vi "Append Image HF.vi"(0 "PDF Report IN":T24(xcontrol), 2 "Header or footer":T1={"Start at page"=1, "H/F Alignment"=enum."CENTER - middle", "Path"=path "", "Image (%)"=100.0, "Link"=""}, 11 "error in (no error)":errorcluster, 13 "Position":T3) -> (4 "PDF Report OUT":T24(xcontrol), 15 "error out":errorcluster)   [LabVIEW 2013]
doc: "Appends an <B>image</B> in a column header (or footer). You can use this polymorphic VI to append a colomn to a header (or footer). The data type you wire to the <B>Header or footer</B> input determines the polymorphic instance to use.\n\nThe header (or footer) can be divided up into three columns. Each column has the same width. The number of header (or footer) that you add determines the number of columns.\n\n<B>FRANÇAIS</B>\nAjoute une <B>image</B> dans une colonne d'un en-tête (ou d'un pied de page). Vous pouvez utiliser ce VI polymorphique pour ajouter une colonne à un en-tête (ou un pied de page). Le type de variable que vous reliez au terminal <B>Header or footer</B> détermine l'instance polymorphique à utiliser.\n\nL'en-tête (ou le pied de page) peut être divisé en un maximum de trois colonnes. Chaque colonne a la même largeur. Le nombre d'en-têtes (ou de pieds de page) que vous ajoutez détermine le nombre de colonnes.\n\n\n\nVersion 1.0\nDeveloped by Jean-Marc Simard\nCopyright © 2010, Exaprom Inc.\nAll rights reserved.\nLicense: BSD\n\nWith iTextSharp 4.1.6 (http://itextsharp.sourceforge.net)\nunder Mozilla Public License Version 1.1\n(http://www.mozilla.org/MPL/MPL-1.1.html)"
uses:
  Controls/PDF Report Xcontrol/PDF Report.xctl
  Controls/Header or Footer.ctl
  Controls/Header or Footer  Image cluster.ctl
  Controls/H F Alignment.ctl
  Controls/Header Footer cluster.ctl
  Controls/Header Footer Type.ctl
  Controls/Header footer horiz alignment.ctl
  Controls/Cell Vertical alignment.ctl
  Controls/Page number.ctl
  Controls/Font cluster.ctl
  Controls/Font size.ctl
  Controls/Font color.ctl
  Controls/Header Footer Line.ctl
  C:/Users/MaxCorp/Documents/GitHub/TopView/DLL/itextsharp.dll
  DLL/itextsharp.dll
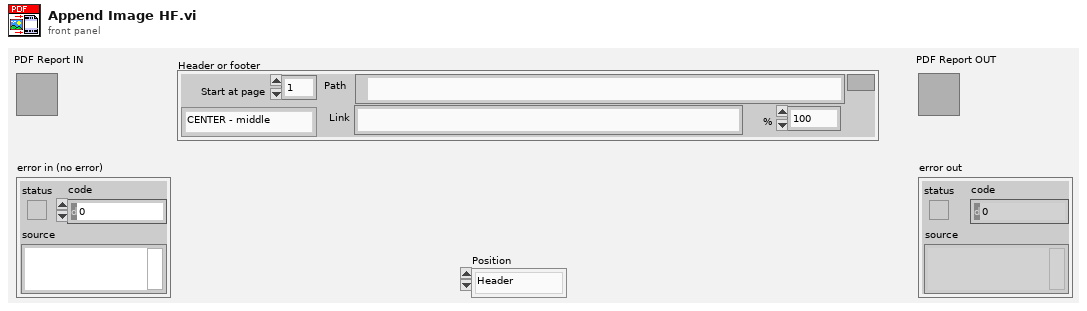
[diagram p1: front panel]
types:
  T1 = typedef "Header or Footer  Image cluster.ctl" = cluster{"Start at page":i32, "H/F Alignment":T2, "Path":path, "Image (%)":sgl, "Link":string}
  T2 = typedef "H F Alignment.ctl" = enum16{"LEFT - top", "LEFT - middle", "LEFT - bottom", "CENTER - top", "CENTER - middle", "CENTER - bottom", "RIGHT - top", "RIGHT - middle", "RIGHT - bottom", ""}
  T3 = typedef "Header or Footer.ctl" = enum16{"Header", "Footer"}
  T4 = typedef "Font cluster.ctl" = cluster{"Name":string, "Size":T5, "Color":T6, "Style":cluster{"Bold":bool, "Italic":bool, "Underline":bool, "Strikeout":bool}}
  T5 = typedef "Font size.ctl" = sgl
  T6 = typedef "Font color.ctl" = u32
  T7 = typedef "Unit.ctl" = enum16{"inch", "mm"}
  T8 = typedef "Paragraphe cluster.ctl" = cluster{" Aligment":T9, "Line spacing":T10}
  T9 = typedef "Texte alignement.ctl" = enum16{"Select", "CENTER", "JUSTIFY", "LEFT", "RIGHT"}
  T10 = typedef "Line spacing.ctl" = enum16{"Select", "1.0", "1.5", "2.0"}
  T11 = typedef "Page dimensions.ctl" = cluster{"Start at page":i32, "Orientation":T12, "widht":sgl, "height":sgl, "Margin left":sgl, "Margin right":sgl, "Margin top":sgl, "Margin bottom":sgl}
  T12 = typedef "Page Orientation.ctl" = enum16{"Portrait", "Landscape"}
  T13 = typedef "Image or Table Caption.ctl" = cluster{"Caption":string, "Separator":string, "Position":enum16{"Above", "Below"}}
  T14 = typedef "Header Footer [ ].ctl" = T15[]
  T15 = typedef "Header Footer cluster.ctl" = cluster{"Start page":i32, "Type":T16, "Alignment":T17, "Vertical Alignement":T18, "Image (%)":sgl, "Page #":T19, "Text":string, "Path":string, "Font":T4, "Font refnum":refnum<k24>, "Line":cluster{"Line":T20, "Thickness (points)":sgl, "Colour":T6}}
  T16 = typedef "Header Footer Type.ctl" = enum16{"Select", "Text", "Text + hyperlink", "Page number", "Image", "Image + hyperlink"}
  T17 = typedef "Header footer horiz alignment.ctl" = enum16{"Left", "Center", "Right"}
  T18 = typedef "Cell Vertical alignment.ctl" = enum16{"TOP", "MIDDLE", "BOTTOM"}
  T19 = typedef "Page number.ctl" = cluster{"Text 1":string, "Text 2":string, "Text 3":string}
  T20 = typedef "Header Footer Line.ctl" = enum16{"No line", "Horizontal line"}
  T21 = typedef "Watermark cluster2.ctl" = cluster{"Show? (F)":bool, "Type":enum16{"Image", "Text"}, "Opacity (%)":sgl, "Rotate(°)":sgl, "Position":cluster{"Position":T22, "X":sgl, "Y":sgl}, "Image path":path, "Scaled(%)":sgl, "Image refnum":refnum<k24>, "Text":string, "Font":cluster{"Name":string, "Size":T5, "Color":T6}, "Font refnum":refnum<k24>, "Alignment":T17, "Automatic":bool}
  T22 = typedef "Watermark Position.ctl" = enum16{"Absolute", "Center (page)", "Center (text section)"}
  T23 = typedef "System Fonts.ctl" = cluster{"Font name [ ]":string[], "Font and file names [ ]":cluster{"Font name":string, "File name":string}[]}
  T24 = cluster{"Document":refnum<k24>, "Writer":refnum<k24>, "Default Font":refnum<k24>, "Default Font cluster":T4, "Path":path, "Unit (default = mm)":T7, "Paragraphe cluster":T8, "Pages dimensions [ ]":T11[], "Captions":cluster{"Image":T13, "Image counter":u16, "Table":T13, "Table counter":u16, "Font":T4}, "Header":T14, "Footer":T14, "Watermark ":T21, "Actual VI name":string, "System Fonts":T23}
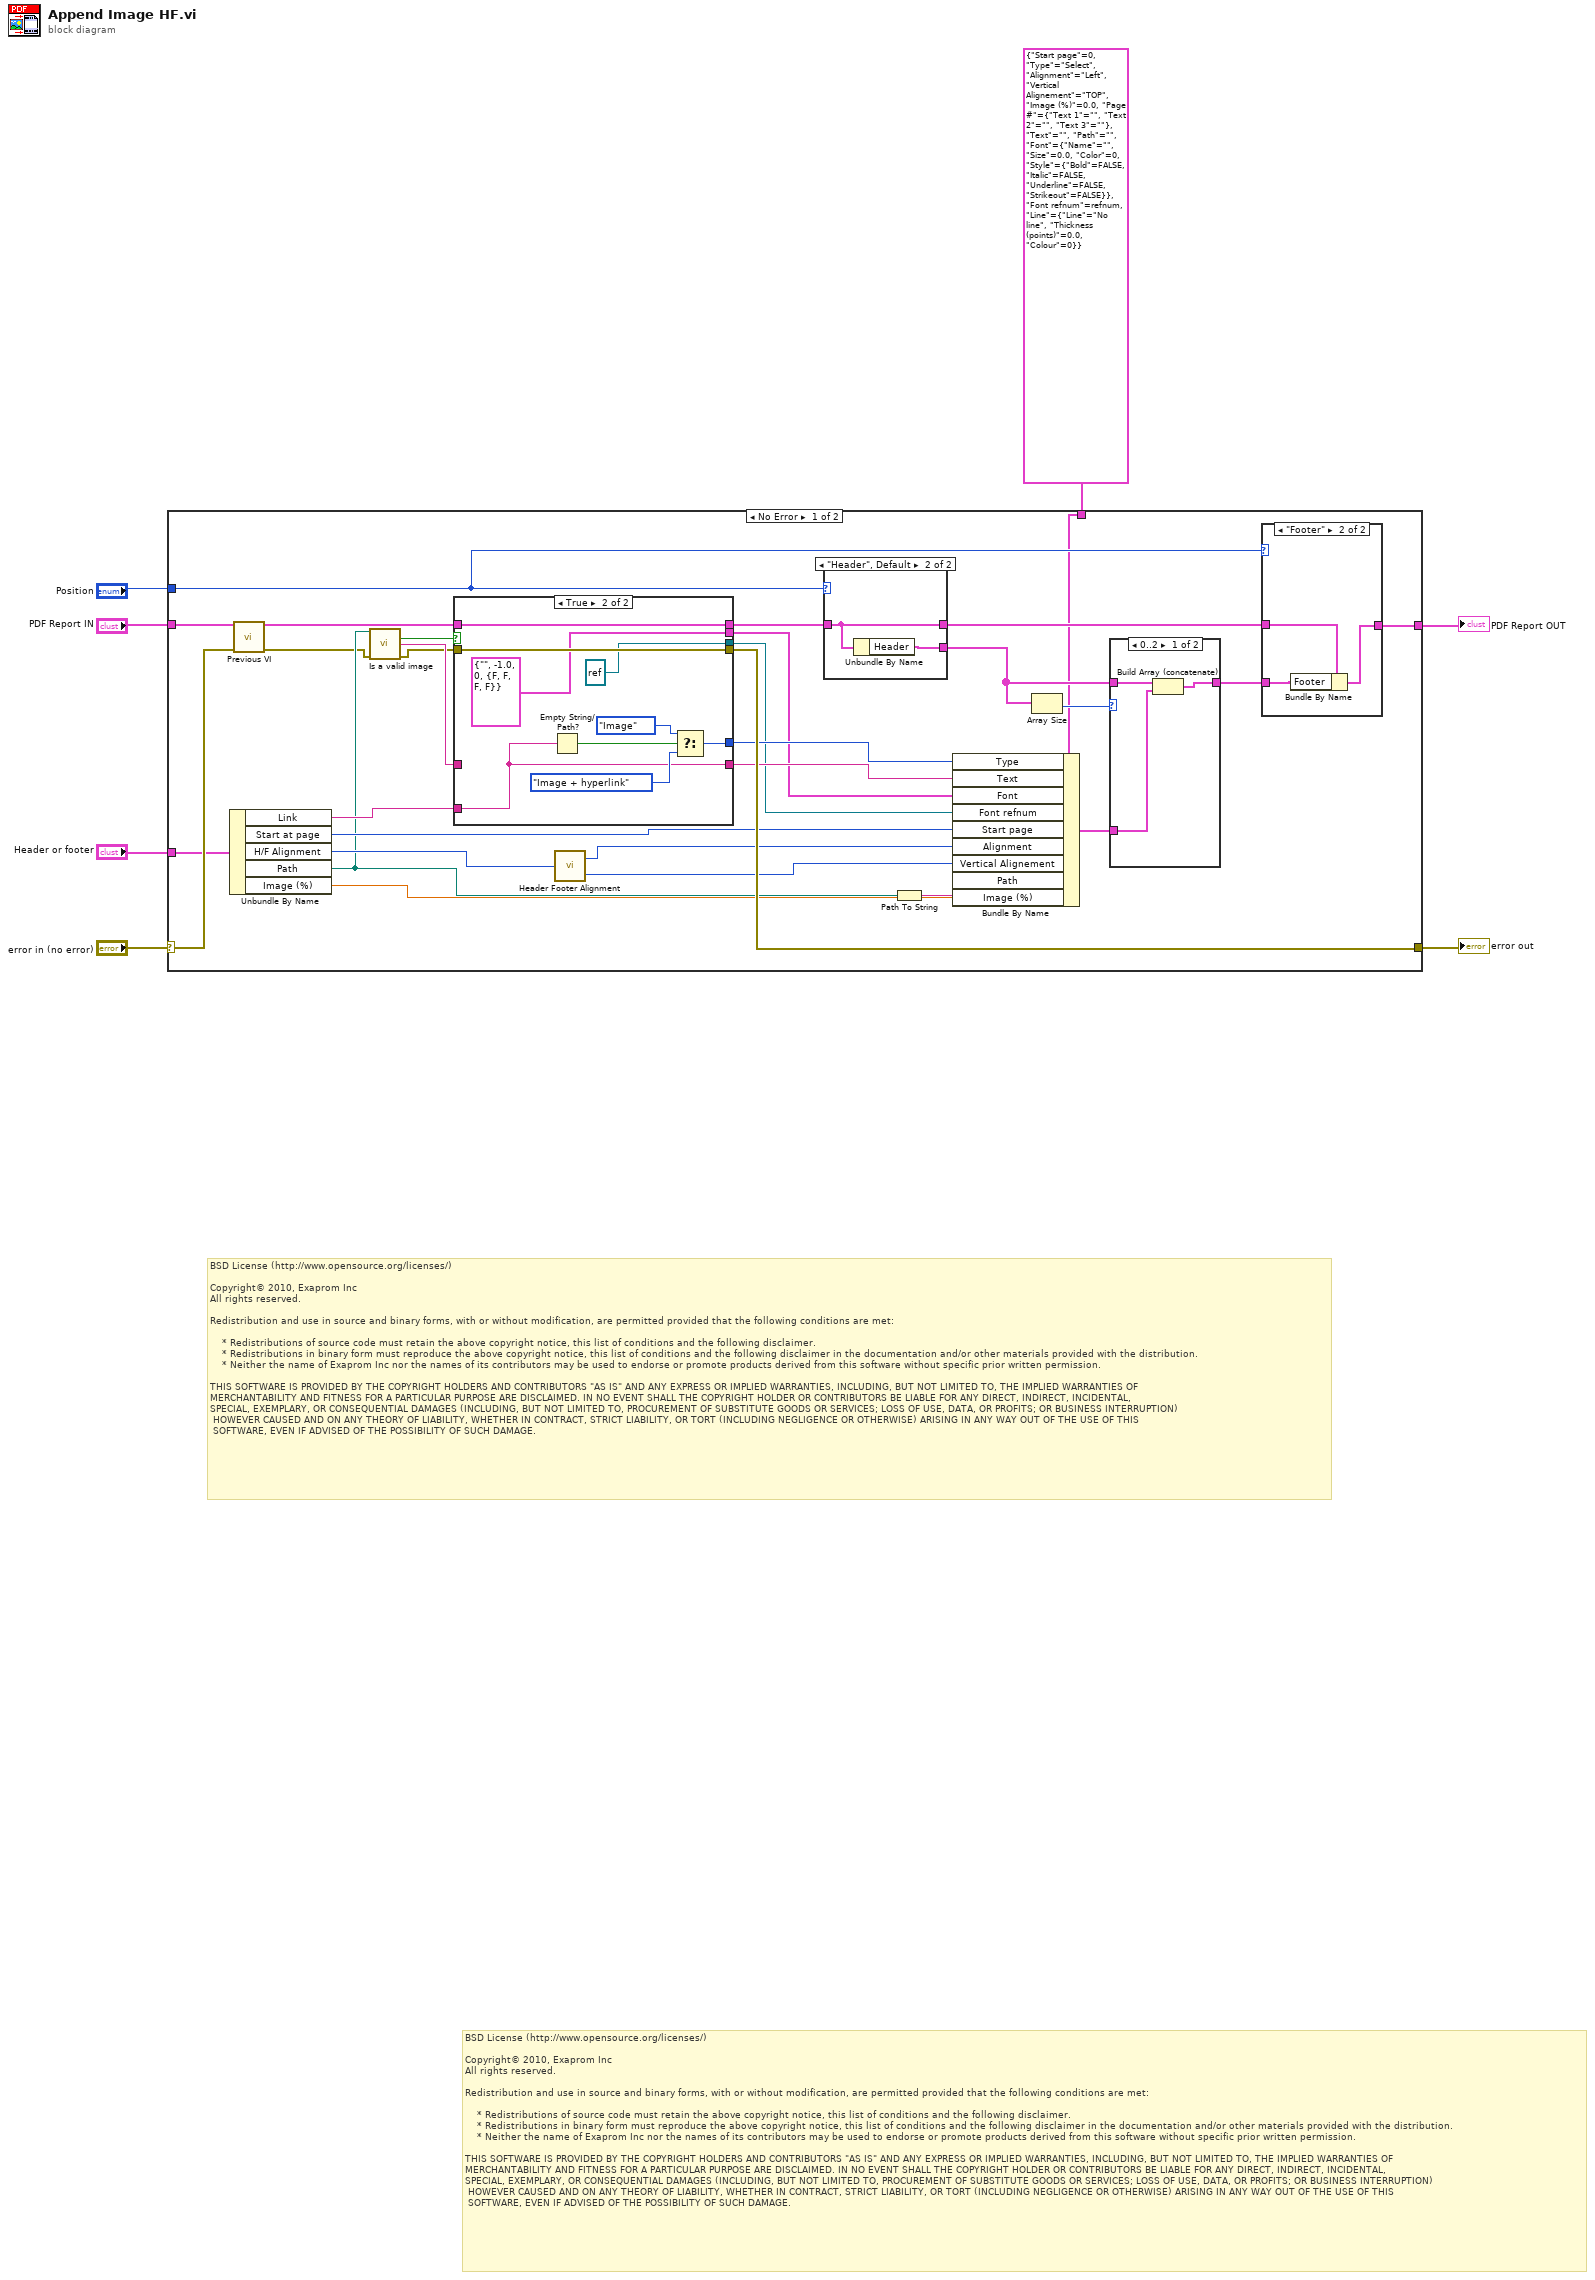
[diagram p0: block diagram]
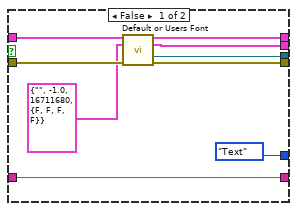
[diagram p2: hidden frame]
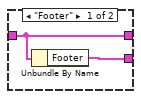
[diagram p4: hidden frame]
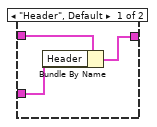
[diagram p5: hidden frame]
diagram:
  # "BSD License (http://www.opensource.org/licenses/)\n\nCopyright© 2010, Exaprom Inc\nAll rights reserved.\n\nRedistribution and use in source and binary forms, with or without modification, are permitted provided that the following conditions are met:\n\n    * Redistributions of source code must retain the above copyright notice, this list of conditions and the following disclaimer.\n    * Redistributions in binary form must reproduce the above copyright notice, this list of conditions and the following disclaimer in the documentation and/or other materials provided with the distribution.\n    * Neither the name of Exaprom Inc nor the names of its contributors may be used to endorse or promote products derived from this software without specific prior written permission.\n\nTHIS SOFTWARE IS PROVIDED BY THE COPYRIGHT HOLDERS AND CONTRIBUTORS \"AS IS\" AND ANY EXPRESS OR IMPLIED WARRANTIES, INCLUDING, BUT NOT LIMITED TO, THE IMPLIED WARRANTIES OF \nMERCHANTABILITY AND FITNESS FOR A PARTICULAR PURPOSE ARE DISCLAIMED. IN NO EVENT SHALL THE COPYRIGHT HOLDER OR CONTRIBUTORS BE LIABLE FOR ANY DIRECT, INDIRECT, INCIDENTAL,\nSPECIAL, EXEMPLARY, OR CONSEQUENTIAL DAMAGES (INCLUDING, BUT NOT LIMITED TO, PROCUREMENT OF SUBSTITUTE GOODS OR SERVICES; LOSS OF USE, DATA, OR PROFITS; OR BUSINESS INTERRUPTION)\n HOWEVER CAUSED AND ON ANY THEORY OF LIABILITY, WHETHER IN CONTRACT, STRICT LIABILITY, OR TORT (INCLUDING NEGLIGENCE OR OTHERWISE) ARISING IN ANY WAY OUT OF THE USE OF THIS\n SOFTWARE, EVEN IF ADVISED OF THE POSSIBILITY OF SUCH DAMAGE."
  # "BSD License (http://www.opensource.org/licenses/)\n\nCopyright© 2010, Exaprom Inc\nAll rights reserved.\n\nRedistribution and use in source and binary forms, with or without modification, are permitted provided that the following conditions are met:\n\n    * Redistributions of source code must retain the above copyright notice, this list of conditions and the following disclaimer.\n    * Redistributions in binary form must reproduce the above copyright notice, this list of conditions and the following disclaimer in the documentation and/or other materials provided with the distribution.\n    * Neither the name of Exaprom Inc nor the names of its contributors may be used to endorse or promote products derived from this software without specific prior written permission.\n\nTHIS SOFTWARE IS PROVIDED BY THE COPYRIGHT HOLDERS AND CONTRIBUTORS \"AS IS\" AND ANY EXPRESS OR IMPLIED WARRANTIES, INCLUDING, BUT NOT LIMITED TO, THE IMPLIED WARRANTIES OF \nMERCHANTABILITY AND FITNESS FOR A PARTICULAR PURPOSE ARE DISCLAIMED. IN NO EVENT SHALL THE COPYRIGHT HOLDER OR CONTRIBUTORS BE LIABLE FOR ANY DIRECT, INDIRECT, INCIDENTAL,\nSPECIAL, EXEMPLARY, OR CONSEQUENTIAL DAMAGES (INCLUDING, BUT NOT LIMITED TO, PROCUREMENT OF SUBSTITUTE GOODS OR SERVICES; LOSS OF USE, DATA, OR PROFITS; OR BUSINESS INTERRUPTION)\n HOWEVER CAUSED AND ON ANY THEORY OF LIABILITY, WHETHER IN CONTRACT, STRICT LIABILITY, OR TORT (INCLUDING NEGLIGENCE OR OTHERWISE) ARISING IN ANY WAY OUT OF THE USE OF THIS\n SOFTWARE, EVEN IF ADVISED OF THE POSSIBILITY OF SUCH DAMAGE."
  n1 = case shown="No Error" "error in (no error)" {
    selector: "error in (no error)" -> [w27 w71]
    tunnel: "PDF Report IN" -> [w35 w70]
    tunnel: "Position" -> [w33 _]
    tunnel: [w36 w70] -> w3
    tunnel: [w37 w71] -> w2
    tunnel: "Header or footer" -> [w26 _]
    tunnel: T15 {"Start page"=0, "Type"=enum."Select", "Alignment"=enum."Left", "Vertical Alignement"=enum."TOP", "Image (%)"=0.0, "Page #"={"Text 1"="", "Text 2"="", "Text 3"=""}, "Text"="", "Path"="", "Font"={"Name"="", "Size"=0.0, "Color"=0, "Style"={"Bold"=FALSE, "Italic"=FALSE, "Underline"=FALSE, "Strikeout"=FALSE}}, "Font refnum"=refnum, "Line"={"Line"=enum."No line", "Thickness (points)"=0.0, "Colour"=0}} ("element") -> [w28 _]
    frame No Error {
      n2 = Unbundle By Name(w26) -> ("Link"=w18:string, "Start at page"=w24:i32, "H/F Alignment"=w21:T2, "Path"=w16:path, "Image (%)"=w19:sgl)
      n3 = call "Previous VI.vi"("PDF Report IN"=w35, "error in (no error)"=w27) -> ("PDF Report OUT"=w14:T24, "error out"=w9:errorcluster)  [unwired: 12 out]
      n4 = call "Is a valid image.vi"("Image path"=w16, "error in (no error)"=w9) -> ("Valid Image?"=w25:bool, "Message"=w17:string, "error out"=w8:errorcluster)  [unwired: 11 out]
      n5 = case shown="True" w25 {
        tunnel: [Header_Footer_Type."Text" ("Type") w54] -> w13
        tunnel: w18 -> [_ w51]
        tunnel: [w45 w51] -> w12
        tunnel: w17 -> [w45 _]
        tunnel: [w43 w50] -> w15
        tunnel: w14 -> [w44 w50]
        tunnel: w8 -> [w42 w49]
        tunnel: [w41 T4 {"Name"="", "Size"=-1.0, "Color"=0, "Style"={"Bold"=FALSE, "Italic"=FALSE, "Underline"=FALSE, "Strikeout"=FALSE}} ("Font OUT")] -> w11
        tunnel: [w40 refnum<k24> refnum ("Font Ref")] -> w10
        tunnel: [w39 w49] -> w37
        frame False {
          n6 = call "Default or Users Font.vi"("PDF Report"=w44, "Font"=T4 {"Name"="", "Size"=-1.0, "Color"=16711680, "Style"={"Bold"=FALSE, "Italic"=FALSE, "Underline"=FALSE, "Strikeout"=FALSE}} ("Font OUT"), "error in (no error)"=w42) -> ("PDF Report duplicate"=w43:T24, "Font OUT"=w41:T4, "Font Ref"=w40:refnum<k24>, "error out"=w39:errorcluster)  [unwired: 9 out]
        }
        frame True {
          n7 = Empty String/Path?(string/path=w51) -> (empty?=w55:bool)
          n8 = Select(t=Header_Footer_Type."Image" ("Type"), s=w55, f=Header_Footer_Type."Image + hyperlink" ("Type")) -> (s? t:f=w54:T16)
        }
      }
      n9 = call "Header Footer Alignment.vi"("H/F Alignment"=w21) -> ("Vertical Alignement"=w22:T18, "Horizontal Alignment"=w23:T17)  [unwired: 2 out]
      n10 = case shown="\"Header\", Default" w33 {
        tunnel: w15 -> [w61 w63]
        tunnel: [w61 w63] -> w34
        tunnel: [w60 w62] -> w29
        frame "Footer" {
          n11 = Unbundle By Name(w61) -> ("Footer"=w60:T14)
        }
        frame "Header", Default {
          n12 = Unbundle By Name(w63) -> ("Header"=w62:T14)
        }
      }
      n13 = Path To String(path=w16) -> (string=w20:string)
      n14 = Bundle By Name(cluster=w28, "Type"=w13, "Text"=w12, "Font"=w11, "Font refnum"=w10, "Start page"=w24, "Alignment"=w23, "Vertical Alignement"=w22, "Path"=w20, "Image (%)"=w19) -> (w32:T15)
      n15 = Array Size(array=w29) -> (size(s)=w30:i32)
      n16 = case shown="0..2" w30 {
        tunnel: w32 -> [w58 _]
        tunnel: [w56 w59] -> w31
        tunnel: w29 -> [w57 w59]
        frame 0..2 {
          n17 = Build Array (concatenate)(w57, w58) -> (w56:T14)
        }
        frame 3.., Default {
        }
      }
      n18 = case shown="\"Footer\"" w33 {
        tunnel: w34 -> [w66 w69]
        tunnel: w31 -> [w64 w67]
        tunnel: [w65 w68] -> w36
        frame "Header", Default {
          n19 = Bundle By Name(cluster=w66, "Header"=w64) -> (w65:T24)
        }
        frame "Footer" {
          n20 = Bundle By Name(cluster=w69, "Footer"=w67) -> (w68:T24)
        }
      }
    }
    frame Error {
    }
  }
  "PDF Report OUT" <- w3
  "error out" <- w2
